vi "AFM_Litho_Plugin.Data.GetPrivateEvents.vi"(8 "error in (no error)":errorcluster, 11 "AFM_Litho_Plugin.Data":refnum<class "AFM_Litho_Plugin.Data.lvclass">) -> (0 "error out":errorcluster, 2 "Private Events":T1, 3 "AFM_Litho_Plugin.Data out":refnum<class "AFM_Litho_Plugin.Data.lvclass">)   [LabVIEW 2019, in "AFM_Litho_Plugin.Data.lvclass"]
doc: "---------------------------------------------------------------\nJKI State Machine Objects™\nhttp://jki.net/state-machine-objects/\nCopyright (C) 2005-2015, JKI <info@jki.net>\nALL RIGHTS RESERVEDJKI State Machine Objects (SMO) 1.0.0.4\nJKI - JKI\nCopyright (c) 2015, JKI"
uses:
  AFM_Litho_Plugin.Data.lvclass
  Typedefs/PrivateEvents--Cluster.ctl
  Typedefs/PrivateEvents--AFM_Litho_Plugin.Data.SaveSweep.ctl
  AFM_Litho_Plugin.Data.lvclass/AFM_Litho_Plugin.Data.ctl
panel:
  # "For instructions on how to use the JKI State Machine Objects, examples and video tutorials, visit:\nhttp://jki.net/state-machine-objects/\n\nJKI State Machine Objects™\nhttp://jki.net/state-machine-objects/\nCopyright (C) 2005-2015, JKI <info@jki.net>\nALL RIGHTS RESERVED"
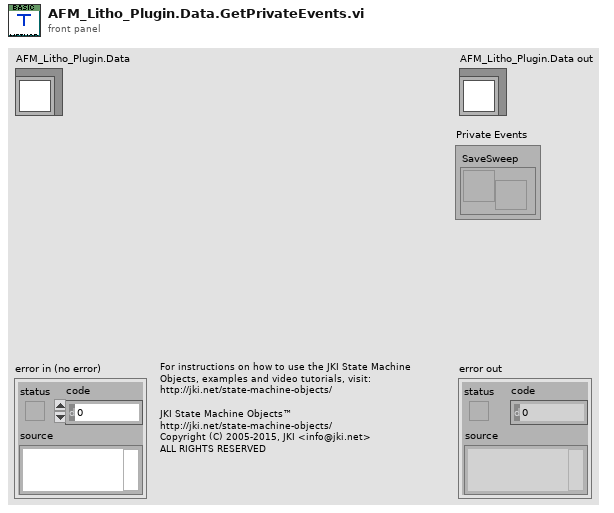
[diagram p1: front panel]
types:
  T1 = typedef "AFM_Litho_Plugin.Data.lvclass/PrivateEvents--Cluster.ctl" = cluster{"SaveSweep":refnum<user-event>}
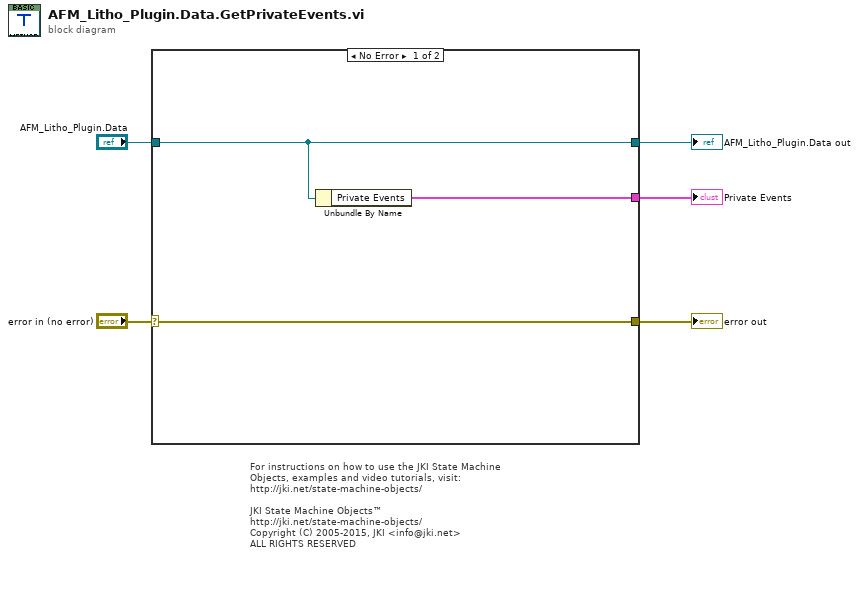
[diagram p0: block diagram]
diagram:
  # "For instructions on how to use the JKI State Machine Objects, examples and video tutorials, visit:\nhttp://jki.net/state-machine-objects/\n\nJKI State Machine Objects™\nhttp://jki.net/state-machine-objects/\nCopyright (C) 2005-2015, JKI <info@jki.net>\nALL RIGHTS RESERVED"
  n1 = case shown="No Error" "error in (no error)" {
    selector: "error in (no error)" -> [w7 w9]
    tunnel: "AFM_Litho_Plugin.Data" -> [w6 w10]
    tunnel: [w7 w9] -> w4
    tunnel: [w6 w10] -> w3
    tunnel: [w8 _] -> w1
    frame No Error {
      n2 = Unbundle By Name(w6) -> ("Private Events"=w8:T1)
    }
    frame Error {
    }
  }
  "error out" <- w4
  "AFM_Litho_Plugin.Data out" <- w3
  "Private Events" <- w1
